vi "MPExxx_Conf_example.vi"() -> ()   [LabVIEW 2012]
doc: "This VI form sets the configuration of the supply."
panel:
  out "error out":errorcluster
  in  "error in (no error)":errorcluster
  in  "Interlock":bool
  in  "External Control":bool
  in  "Internal Control":bool=TRUE
  in  "Remote Sense":bool
  in  "OCP":dbl format="%.2f"
  in  "OVP":dbl format="%.2f"
  in  "Current":dbl format="%.2f"
  in  "Voltage":dbl format="%.2f"
  in  "VISA Resource Name":refnum<visa-resource-name>
  # "MAGNA-POWER"
  # "Electronics"
  # "Instrument Settings"
  # "Configuration Settings"
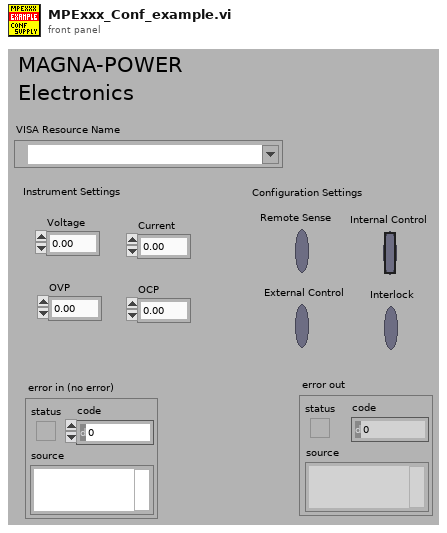
[diagram p1: front panel]
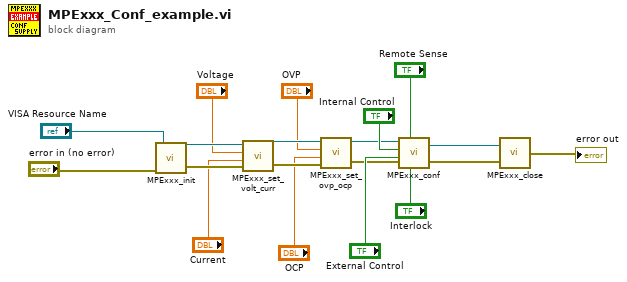
[diagram p0: block diagram]
diagram:
  n1 = call "MPExxx_init.vi"("error in (no error)"="error in (no error)", "VISA session"="VISA Resource Name") -> ("error out"=w18:errorcluster, "dup VISA session"=w15:refnum<visa-resource-name>)  [unwired: 2 in]
  n2 = call "MPExxx_set_volt_curr.vi"("error in (no error)"=w18, "Set Current"="Current", "Set Voltage"="Voltage", "VISA session"=w15) -> ("error out"=w17:errorcluster, "dup VISA session"=w16:refnum<visa-resource-name>)
  n3 = call "MPExxx_set_ovp_ocp.vi"("error in (no error)"=w17, "Set OCP"="OCP", "Set OVP"="OVP", "VISA session"=w16) -> ("error out"=w3:errorcluster, "dup VISA session"=w4:refnum<visa-resource-name>)
  n4 = call "MPExxx_conf.vi"("Interlock"="Interlock", "Remote Sense"="Remote Sense", "error in (no error)"=w3, "External Control"="External Control", "Internal Control"="Internal Control", "VISA session"=w4) -> ("error out"=w2:errorcluster, "dup VISA session"=w1:refnum<visa-resource-name>)
  n5 = call "MPExxx_close.vi"("error in (no error)"=w2, "VISA session"=w1) -> ("error out"=→"error out":errorcluster)
